vi "Checksum.vi"(2 "Invert (F)":bool, 3 "String":string, 4 "Type (0)":u32(ring) items=["XOR", "8 bit sum (MOD 100h)", "8 bit LRC", "16 bit sum (MOD 10000h)", "MODBUS CRC 16 bit", "XOR 16 bit"]) -> (0 "Checksum hex":string, 1 "Checksum dec":string)   [LabVIEW 2014]
doc: "Checksum.vi\nComputes checksum\n\nType (0) - Checksum type\n 0: XOR of characters (8 bit)\n 1: Modulo 100h of sum of characters (8 bit sum)\n 2: LRC (8 bit), 256 - Modulo 100h of sum of characters\n 3: Modulo 10000h of sum of characters (16 bit sum)\n 4: MODBUS 16 bit CRC\nString - String to compute checksum from\nInvert (F) - If TRUE inverts checksum result\n\nChecksum dec - Decimal value represented by 1 or 2 ASCII characters (8 bit or 16 bit)\nChecksum hex - Hex value represented by 2 or 4 ASCII characters (8 bit or 16 bit)\n\nLM"
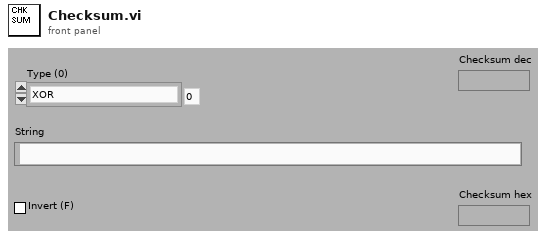
[diagram p1: front panel]
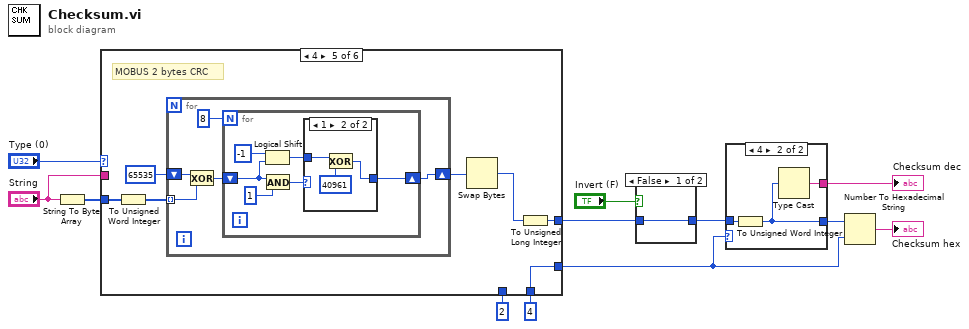
[diagram p0: block diagram]
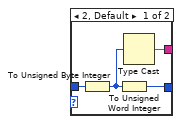
[diagram p2: hidden frame]
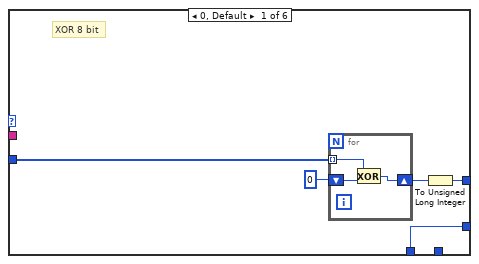
[diagram p3: hidden frame]
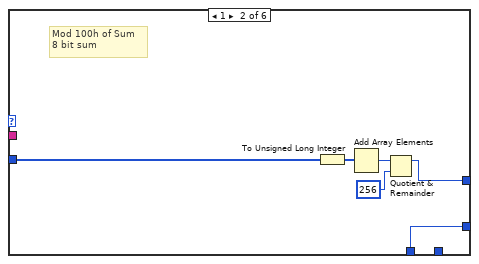
[diagram p4: hidden frame]
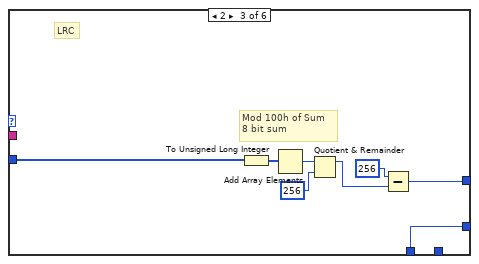
[diagram p5: hidden frame]
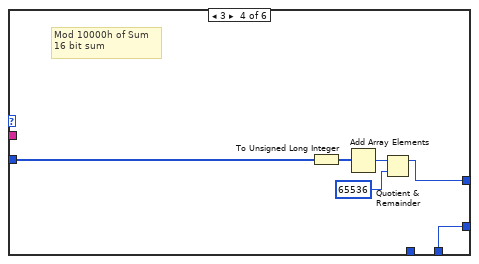
[diagram p6: hidden frame]
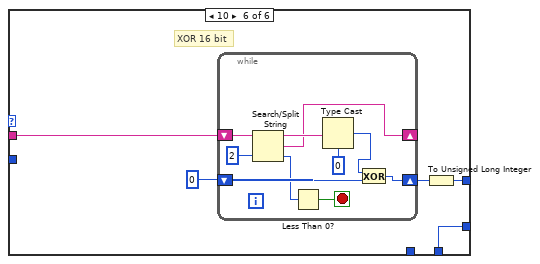
[diagram p8: hidden frame]
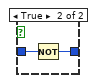
[diagram p9: hidden frame]
diagram:
  n1 = String To Byte Array(string="String") -> (unsigned byte array=w6:u8[])
  n2 = case shown="4" "Type (0)" {
    tunnel: [w14 w22 w28 w36 w43 w66] -> w5
    tunnel: w6 -> [w13 w21 w31 w35 w46 _]
    tunnel: 2 -> [w15 w23 w29 _ _ _]
    tunnel: [w15 w23 w29 w38 w44 w64] -> w8
    tunnel: 4 -> [_ _ _ w38 w44 w64]
    tunnel: "String" -> [_ _ _ _ _ w63]
    frame 0, Default {
      # "XOR 8 bit"
      n3 = for {
        tunnel: w13 -> [w18] mode=indexing
        shift-right: [w19] -> w16
        shift-left: u8 0 -> [w20]
        n4 = Exclusive Or(1:w20, 2:w18) -> (0:w19:u8)
      }
      n5 = To Unsigned Long Integer(number=w16) -> (unsigned 32bit integer=w14:u32)
    }
    frame 1 {
      # "Mod 100h of Sum\n8 bit sum"
      n6 = To Unsigned Long Integer(number=w21) -> (unsigned 32bit integer=w25:u32[])
      n7 = Add Array Elements(numeric array=w25) -> (sum=w24:u32)
      n8 = Quotient & Remainder(x=w24, y=u32 256) -> (x-y*floor(x/y)=w22:u32)  [unwired: 1 out]
    }
    frame 2 {
      # "LRC"
      # "Mod 100h of Sum\n8 bit sum"
      n9 = To Unsigned Long Integer(number=w31) -> (unsigned 32bit integer=w33:u32[])
      n10 = Add Array Elements(numeric array=w33) -> (sum=w32:u32)
      n11 = Quotient & Remainder(x=w32, y=u32 256) -> (x-y*floor(x/y)=w30:u32)  [unwired: 1 out]
      n12 = Subtract(x=u32 256, y=w30) -> (x-y=w28:u32)
    }
    frame 3 {
      # "Mod 10000h of Sum\n16 bit sum"
      n13 = To Unsigned Long Integer(number=w35) -> (unsigned 32bit integer=w37:u32[])
      n14 = Add Array Elements(numeric array=w37) -> (sum=w39:u32)
      n15 = Quotient & Remainder(x=w39, y=u32 65536) -> (x-y*floor(x/y)=w36:u32)  [unwired: 1 out]
    }
    frame 4 {
      # "MOBUS 2 bytes CRC"
      n16 = To Unsigned Word Integer(number=w46) -> (unsigned 16bit integer=w45:u16[])
      n17 = for {
        tunnel: w45 -> [w51] mode=indexing
        shift-right: [w48] -> w42
        shift-left: u16 65535 -> [w50]
        n18 = Exclusive Or(1:w51, 2:w50) -> (0:w49:u16)
        n19 = for {
          N: 8 -> [_]
          shift-right: [w53] -> w48
          shift-left: w49 -> [w55]
          n20 = Logical Shift(y=-1, x=w55) -> (x << y=w54:u16)
          n21 = And(x=w55, y=u16 1) -> (x .and. y?=w57:u16)
          n22 = case shown="1" w57 {
            tunnel: [w59 w61] -> w53
            tunnel: w54 -> [w59 w60]
            frame 0, Default {
            }
            frame 1 {
              n23 = Exclusive Or(1:u16 40961, 2:w60) -> (0:w61:u16)
            }
          }
        }
      }
      n24 = Swap Bytes(anything=w42) -> (byte swapped=w41:u16)
      n25 = To Unsigned Long Integer(number=w41) -> (unsigned 32bit integer=w43:u32)
    }
    frame 10 {
      # "XOR 16 bit"
      n26 = while {
        shift-right: [w76] -> w67
        shift-left: u16 0 -> [w77]
        shift-right: [w70] -> _
        shift-left: w63 -> [w74]
        stop <- w68 stop-if-true
        n27 = Search/Split String(string=w74, offset (0)=2) -> (substring before match=w72:string, match + rest of string=w70:string, offset of match=w69:i32)  [unwired: 1 in]
        n28 = Less Than 0?(x=w69) -> (x < 0?=w68:bool)
        n29 = Type Cast(type=u16 0, x=w72) -> (*(type *) &x=w71:u16)
        n30 = Exclusive Or(1:w77, 2:w71) -> (0:w76:u16)
      }
      n31 = To Unsigned Long Integer(number=w67) -> (unsigned 32bit integer=w66:u32)
    }
  }
  n32 = case shown="False" "Invert (F)" {
    tunnel: w5 -> [w78 w80]
    tunnel: [w78 w79] -> w7
    frame False {
    }
    frame True {
      n33 = Not(x=w80) -> (.not. x?=w79:u32)
    }
  }
  n34 = case shown="4" w8 {
    tunnel: w7 -> [w84 w87]
    tunnel: [w83 w86] -> w2
    tunnel: [w81 w85] -> w1
    frame 2, Default {
      n35 = To Unsigned Byte Integer(number=w84) -> (unsigned 8bit integer=w82:u8)
      n36 = To Unsigned Word Integer(number=w82) -> (unsigned 16bit integer=w83:u16)
      n37 = Type Cast(x=w82) -> (*(type *) &x=w81:string)  [unwired: 1 in]
    }
    frame 4 {
      n38 = To Unsigned Word Integer(number=w87) -> (unsigned 16bit integer=w86:u16)
      n39 = Type Cast(x=w86) -> (*(type *) &x=w85:string)  [unwired: 1 in]
    }
  }
  "Checksum dec" <- w1
  n40 = Number To Hexadecimal String(1:w8, 2:w2) -> (0:→"Checksum hex":string)
